vi "bytes to read.vi"(1 "Items":u16=10, 2 "Data Type":T1=enum."String") -> (0 "Bytes to read":i32)   [LabVIEW 2014, in "Simatic S7.lvlib"]
uses:
  Simatic S7.lvlib
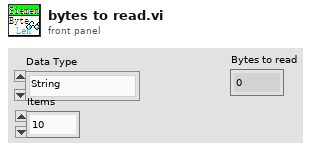
[diagram p1: front panel]
types:
  T1 = typedef "Data Type.ctl" = enum8{"Bit", "Byte (U8)", "Signed Byte (I8)", "Word (U16)", "Signed Word (I16)", "Long (U32)", "Signed Long (I32)", "Real (SGL)", "String"}
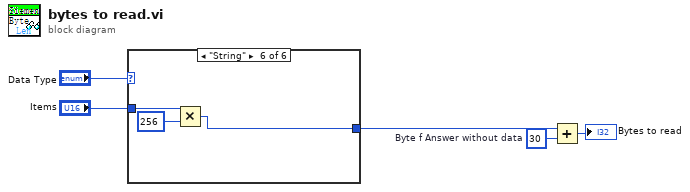
[diagram p0: block diagram]
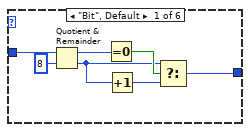
[diagram p2: hidden frame]
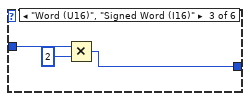
[diagram p4: hidden frame]
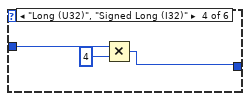
[diagram p5: hidden frame]
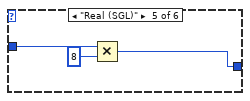
[diagram p6: hidden frame]
diagram:
  w1 = 30  # Byte f Answer without data
  n1 = case shown="\"String\"" "Data Type" {
    tunnel: "Items" -> [w12 w13 w16 w18 w21 w25]
    tunnel: [w6 w13 w14 w17 w20 w23] -> w3
    frame "Bit", Default {
      n2 = Quotient & Remainder(x=w12, y=8) -> (x-y*floor(x/y)=w10:i32, floor(x/y)=w8:i32)
      n3 = Equal To 0?(x=w10) -> (x = 0?=w9:bool)
      n4 = Increment(x=w8) -> (x+1=w7:i32)
      n5 = Select(t=w8, s=w9, f=w7) -> (s? t:f=w6:i32)
    }
    frame "Byte (U8)", "Signed Byte (I8)" {
    }
    frame "Word (U16)", "Signed Word (I16)" {
      n6 = Multiply(x=w16, y=2) -> (x*y=w14:i32)
    }
    frame "Long (U32)", "Signed Long (I32)" {
      n7 = Multiply(x=w18, y=4) -> (x*y=w17:i32)
    }
    frame "Real (SGL)" {
      n8 = Multiply(x=w21, y=8) -> (x*y=w20:i32)
    }
    frame "String" {
      n9 = Multiply(x=w25, y=256) -> (x*y=w23:i32)
    }
  }
  n10 = Add(x=w3, y=w1) -> (x+y=→"Bytes to read":i32)
